vi "SDSU_ExpStatusLoop.vi"(4 "stop ref":refnum<vi>, 6 "exptime":dbl, 7 "Total Phys Buffers":u32, 8 "error in (no error)":errorcluster, 9 "frames command":string, 10 "notifier":refnum<notifier>, 11 "fd":i32) -> (0 "error out":errorcluster, 2 "notifier  out":refnum<notifier>, 3 "fd out":i32)   [LabVIEW 2016]
uses:
  Common/public/vis/CMN_FVAR_action.ctl
  DBSHAND/private/vis/DatabaseHand_Element_Set(double).vi
  c/lib/libarcDHE.so
panel:
  out "read prog":i32
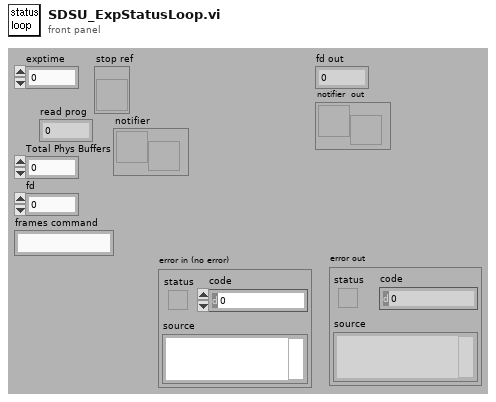
[diagram p1: front panel]
types:
  T1 = typedef "CMN_FVAR_action.ctl" = enum16{"read", "write"}
  T2 = enum16{"Idle", "Exposing", "Paused", "AbortExp", "Reading", "AbortRead", "FinishedReading", "Resetting", "Reducing"}
  T3 = enum16{"Idle", "Exposing", "Paused", "AbortExp", "Reading", "AbortRead", "FinishedReading", "Resetting", "Reducing", "Initializing"}
  T4 = typedef "DatabaseHand_RefNum.ctl" = refnum<vi>
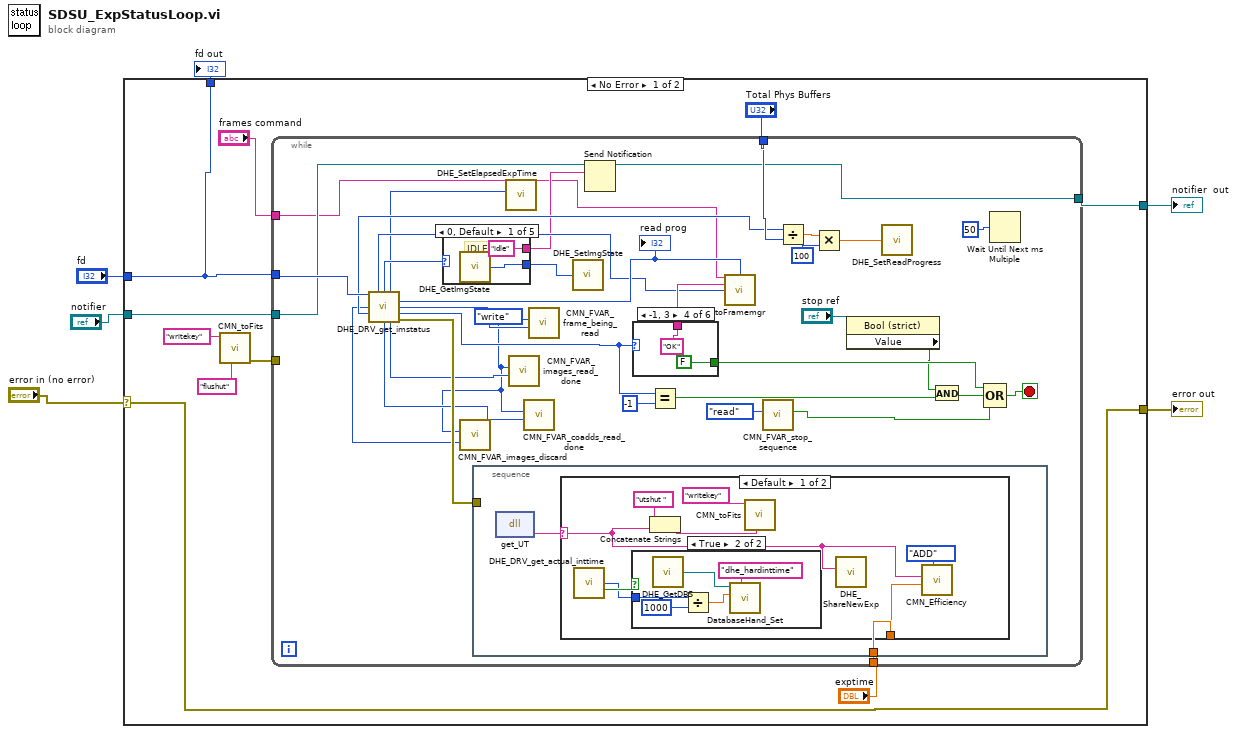
[diagram p0: block diagram]
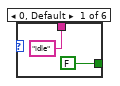
[diagram p4: hidden frame]
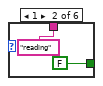
[diagram p5: hidden frame]
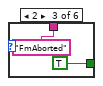
[diagram p6: hidden frame]
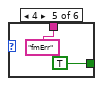
[diagram p7: hidden frame]
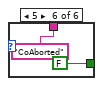
[diagram p8: hidden frame]
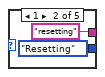
[diagram p9: hidden frame]
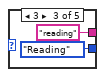
[diagram p10: hidden frame]
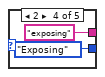
[diagram p11: hidden frame]
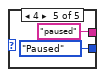
[diagram p12: hidden frame]
diagram:
  n1 = case shown="No Error" "error in (no error)" {
    selector: "error in (no error)" -> [w10 w88]
    tunnel: "fd" -> [w13 w90]
    tunnel: [w13 w90] -> w5
    tunnel: "notifier" -> [w12 w89]
    tunnel: [w11 w89] -> w3
    tunnel: [w10 w88] -> w1
    frame No Error {
      n2 = call "CMN_toFits.vi"("key"="flushut" ("command"), "command"="writekey") -> ("error out"=w7:errorcluster)  [unwired: 6 in, 3 out]
      n3 = while {
        tunnel: "Total Phys Buffers" -> [w45]
        tunnel: w13 -> [w47]
        tunnel: "exptime" -> [w33]
        tunnel: w12 -> [w32]
        tunnel: [w31] -> w11
        tunnel: "frames command" -> [w19]
        tunnel: w7 -> [_]
        stop <- w40 stop-if-true
        w23 = CMN_FVAR_action."write" ("action")
        n4 = call "DHE_DRV_get_imstatus.vi"("fd"=w47) -> ("ptr to buffer"=w42:u64, "image status"=w46:i16, "exposure progress"=w28:i32, "buff read"=w43:i32, "fowlers_discarded"=w24:i32, "frames read"=w27:i32, "actual_buf_reads"=w41:i32, "frame status"=w38:i32, "coadds done"=w25:i32, "images done"=w26:i32, "error out"=w34:errorcluster)  [unwired: 1 in, 3 out]
        "read prog" <- w43
        n5 = case shown="0, Default" w46 {
          tunnel: [w78 T2."Resetting" ("ImgState") T2."Reading" ("ImgState") T2."Exposing" ("ImgState") T2."Paused" ("ImgState")] -> w29
          tunnel: ["idle" "resetting" "reading" "exposing" "paused"] -> w30
          frame 0, Default {
            # "IDLE"
            n6 = call "DHE_GetImgState.vi"() -> ("DHE_ImgState"=w78:T3)  [unwired: 9 out]
          }
          frame 1 {
          }
          frame 3 {
          }
          frame 2 {
          }
          frame 4 {
          }
        }
        n7 = call "CMN_FVAR_images_discard.vi"("value in"=w24, "action"=w23) -> ()  [unwired: 9 out]
        n8 = stacked-sequence {
          tunnel: w34 -> [_]
          tunnel: w33 -> [w51]
          frame #0 {
            n9 = dll-call lib="home/simager/panview/PAN/Modules/SDSU/private/c/lib/libarcDHE.so" fn="get_UT" label="get_KEYS"() -> ("return type"=w52:string)  [unwired: 3 in, 2 out]
            n10 = case shown="Default" w52 {
              selector: w52 -> [w55 _]
              tunnel: w51 -> [w56 _]
              frame Default {
                n11 = call "DHE_DRV_get_actual_inttime.vi"() -> ("actual inttime"=w53:i32, "supported"=w54:bool)  [unwired: 1 in, 13 out]
                n12 = case shown="True" w54 {
                  tunnel: w53 -> [_ w63]
                  frame False {
                  }
                  frame True {
                    n13 = call "DHE_GetDBS.vi"() -> ("DHE_DBSRef"=w65:T4)  [unwired: 9 out]
                    n14 = Divide(x=w63, y=1000) -> (x/y=w61:dbl)
                    n15 = call-poly "DatabaseHand_Set.vi"("name"="dhe_hardinttime", "value"=w61, "Database RefNum in"=w65) -> ()  [unwired: 5 in, 4 out]
                  }
                }
                n16 = Concatenate Strings("utshut " ("Format String"), w55) -> (w58:string)
                n17 = call "CMN_toFits.vi"("key"=w58, "command"="writekey") -> ()  [unwired: 6 in, 4 out]
                n18 = call "DHE_ShareNewExp.vi"("UT in"=w55) -> ()  [unwired: 1 in, 10 out]
                n19 = call "CMN_Efficiency.vi"("Action"=enum16{"ADD", "CLEAR", "GET"}."ADD", "exptime"=w56, "UTSHUT"=w55) -> ()  [unwired: 1 in, 8 out]
              }
              frame "EMPTY" {
              }
            }
          }
        }
        n20 = call "DHE_SetElapsedExpTime.vi"("ElapsedExpTime"=w28) -> ()  [unwired: 11 out]
        n21 = call "CMN_FVAR_images_read_done.vi"("value in"=w26, "action"=w23) -> ()  [unwired: 9 out]
        n22 = call "CMN_FVAR_coadds_read_done.vi"("value in"=w25, "action"=w23) -> ()  [unwired: 9 out]
        n23 = call "CMN_FVAR_frame_being_read.vi"("value in"=w27, "action"=w23) -> ()  [unwired: 9 out]
        n24 = call "DHE_SetImgState.vi"("DHE_ImgState"=w29) -> ()  [unwired: 9 out]
        n25 = Send Notification(notification=w30, notifier=w32) -> (notifier out=w31:refnum<notifier>)  [unwired: 1 in, 1 out]
        n26 = case shown="-1, 3" w38 {
          tunnel: ["idle" "reading" "FmAborted" "OK" "fmErr" "CoAborted"] -> w44
          tunnel: [FALSE FALSE TRUE FALSE TRUE FALSE] -> w35
          frame 0, Default {
          }
          frame 1 {
          }
          frame 2 {
          }
          frame -1, 3 {
          }
          frame 4 {
          }
          frame 5 {
          }
        }
        n27 = Equal?(x=w38, y=-1) -> (x = y?=w36:bool)
        n28 = call "toFramemgr.vi"("command"=w19, "progress"=w43, "arg"=w44, "bufpointer"=w42) -> ()  [unwired: 5 in, 7 out]
        n29 = call "CMN_FVAR_stop_sequence.vi"("action"=CMN_FVAR_action."read") -> ("value out"=w20:bool)  [unwired: 1 in, 8 out]
        n30 = Divide(x=w41, y=w45) -> (x/y=w49:dbl)
        n31 = Multiply(x=w49, y=100) -> (x*y=w22:dbl)
        n32 = property class="Bool (strict)"(reference="stop ref") -> ("Value"=w17:bool)  [unwired: 1 in, 2 out]
        n33 = call "DHE_SetReadProgress.vi"("ReadProgress"=w22) -> ()  [unwired: 11 out]
        n34 = And(x=w17, y=w36) -> (x .and. y?=w39:bool)
        n35 = Compound Arithmetic op=OR(w35, w39, w20) -> (w40:bool)
        n36 = Wait Until Next ms Multiple(millisecond multiple=u32 50) -> ()  [unwired: 1 out]
      }
    }
    frame Error {
    }
  }
  "fd out" <- w5
  "notifier  out" <- w3
  "error out" <- w1
